vi "gwyscan save gwyddion arrays general.vi"(0 "data":dbl, 1 "nchannels":i32, 2 "xres":i32, 3 "yres":i32, 4 "xreal":dbl, 5 "yreal":dbl, 6 "xyunit":string, 7 "error in (no error)":errorcluster, 8 "zunit":string, 9 "description":string, 10 "filename":string) -> (16 "filename out":string, 18 "zunit out":string, 19 "description out":string, 20 "data out":dbl, 21 "function return":i32, 22 "xres out":i32, 23 "yres out":i32, 24 "xreal out":dbl, 25 "yreal out":dbl, 26 "xyunit out":string, 27 "error out":errorcluster)   [LabVIEW 2016, in "libgwyscan.lvlib"]
doc: "GWYSCANDLL_API int gwyscan_save_gwyddion_arrays_general(double **data, int nchannels, int *xres, int *yres, double *xreal, double *yreal, char **xyunit, char **zunit, char **description, char *filename);"
uses:
  libgwyscan.lvlib
  libgwyscan.dll
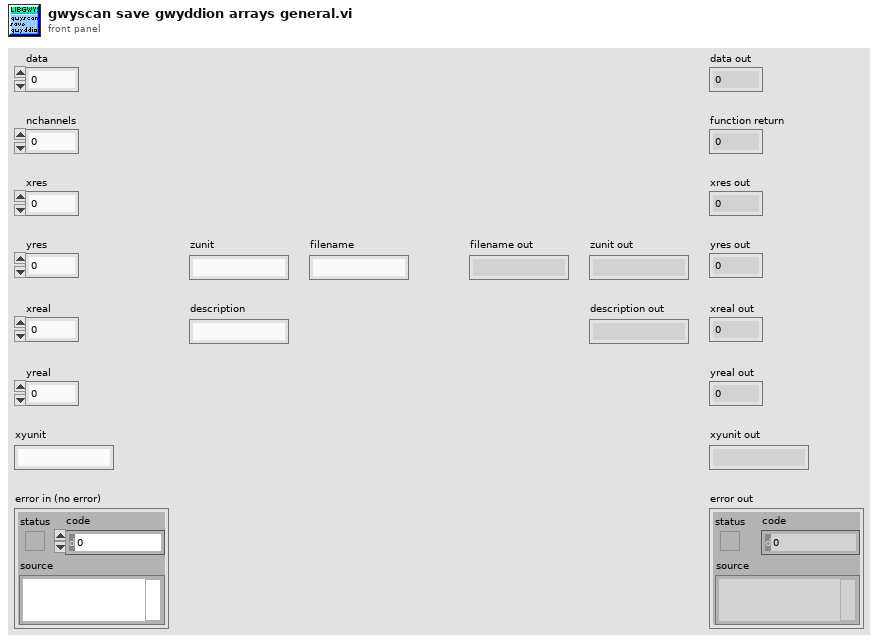
[diagram p1: front panel]
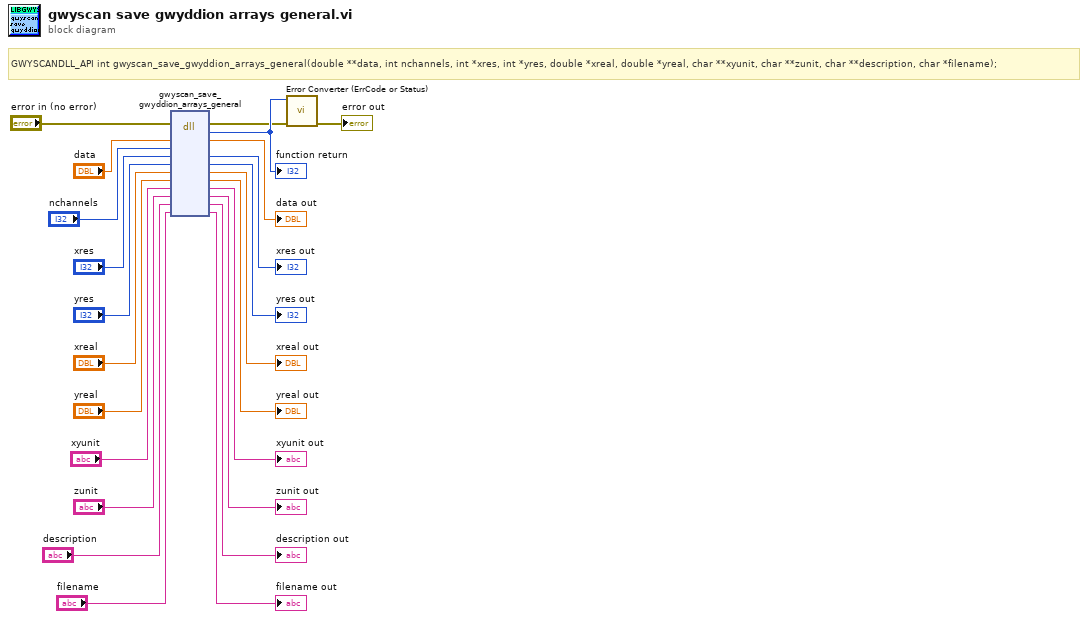
[diagram p0: block diagram]
diagram:
  # "GWYSCANDLL_API int gwyscan_save_gwyddion_arrays_general(double **data, int nchannels, int *xres, int *yres, double *xreal, double *yreal, char **xyunit, char **zunit, char **description, char *filename);"
  n1 = dll-call lib="PTH2abs CUsersCharlÃ¨ne BrillardDesktoplbni-lbniAFMController-BetaVersionv2.0.16-20190611 libgwyscan-1.2-labview2015-win32libgwyscan.*" fn="gwyscan_save_gwyddion_arrays_general"(error in="error in (no error)", "data"="data", "nchannels"="nchannels", "xres"="xres", "yres"="yres", "xreal"="xreal", "yreal"="yreal", "xyunit"="xyunit", "zunit"="zunit", "description"="description", "filename"="filename") -> (error out=w2:errorcluster, w23:i32, "data"=→"data out":dbl, "xres"=→"xres out":i32, "yres"=→"yres out":i32, "xreal"=→"xreal out":dbl, "yreal"=→"yreal out":dbl, "xyunit"=→"xyunit out":string, "zunit"=→"zunit out":string, "description"=→"description out":string, "filename"=→"filename out":string)  [unwired: 3 in, 1 out]
  "function return" <- w23
  n2 = call "Error Converter (ErrCode or Status).vi"("error in (no error)"=w2, "error code"=w23) -> ("error out"=→"error out":errorcluster)  [unwired: 9 in]
